vi "RandomNumbers.vi"() -> ()   [LabVIEW 2020]
panel:
  in  "ms":u32
  out "Signalverlaufsdiagramm":dbl(graph)
  in  "Stopp":bool
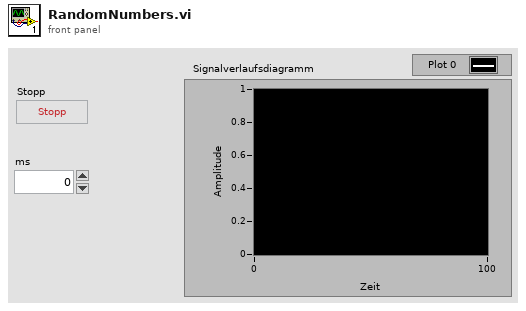
[diagram p1: front panel]
types:
  T1 = enum32{"invalid app kind", "Development System", "Run Time System", "Student Edition", "Embedded LabVIEW", "Evaluation", "Custom"}
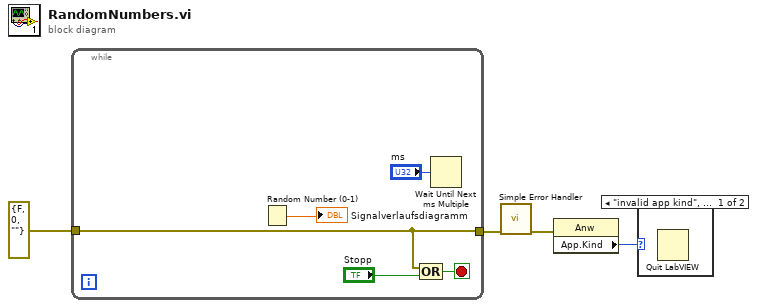
[diagram p0: block diagram]
diagram:
  n1 = while {
    tunnel: errorcluster {"status"=FALSE, "code"=0, "source"=""} ("error in (no error)") -> [w6]
    tunnel: [w6] -> w3
    stop <- w5 stop-if-true
    n2 = Random Number (0-1)() -> (number: 0 to 1=→"Signalverlaufsdiagramm":dbl)
    n3 = Compound Arithmetic op=OR ("Mehrfacharithmetik")(w6, "Stopp") -> (w5:bool)
    n4 = Wait Until Next ms Multiple(millisecond multiple="ms") -> ()  [unwired: 1 out]
  }
  n5 = call <vilib>:"Simple Error Handler.vi"("error in (no error)"=w3) -> ("error out"=w2:errorcluster)  [unwired: 4 in, 4 out]
  n6 = property class="Anw"(error in=w2) -> ("App.Kind"=w1:T1)  [unwired: 1 in, 2 out]
  n7 = case shown="\"invalid app kind\", Standard" w1 {
    frame "invalid app kind", Default {
      n8 = Quit LabVIEW() -> ()  [unwired: 1 in]
    }
    frame "Development System" {
    }
  }
